vi "ROS_Master_getPublishedTopicsReply.vi"(2 "Subgraph":string, 3 "ROS_Master":T1) -> (0 "XML":string)   [LabVIEW 2014]
doc: "Returns the XML reply for a published topic"
uses:
  <userlib>/ROS for LabVIEW Software/ROS/Code/ROS_Master/ROS_Master.ctl
  <userlib>/ROS for LabVIEW Software/ROS/Code/ROS_Master/ROS_Topic.ctl
  <userlib>/ROS for LabVIEW Software/ROS/Code/ROS_Master/ROS_Node.ctl
  <userlib>/ROS for LabVIEW Software/ROS/Code/ROS_Master/ROS_Service.ctl
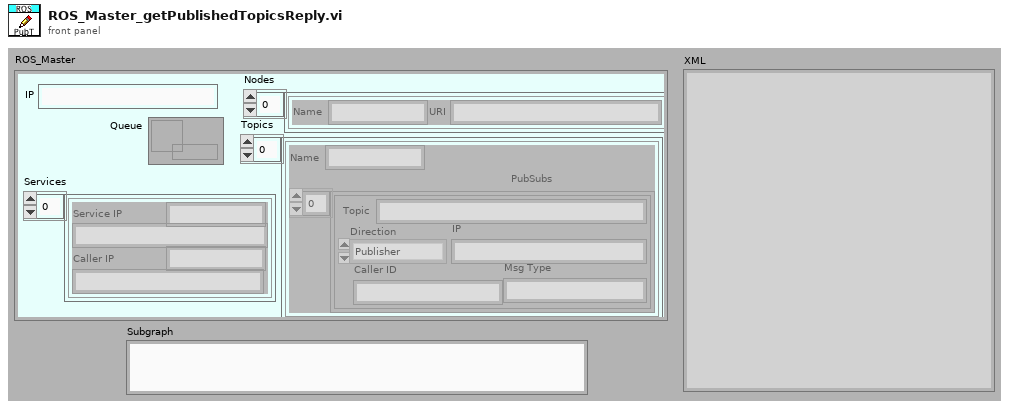
[diagram p1: front panel]
types:
  T1 = typedef "ROS_Master.ctl" = cluster{"IP":string, "Topics":cluster{"Name":string, "PubSubs":T2[]}[], "Nodes":T3[], "Services":T4[], "Queue":refnum<queue>}
  T2 = typedef "ROS_Topic.ctl" = cluster{"Caller ID":string, "IP":string, "Msg Type":string, "Direction":enum16{"Publisher", "Subscriber"}, "Topic":string}
  T3 = typedef "ROS_Node.ctl" = cluster{"Name":string, "URI":string}
  T4 = typedef "ROS_Service.ctl" = cluster{"Service":string, "Service IP":string, "Caller IP":string, "Caller ID":string}
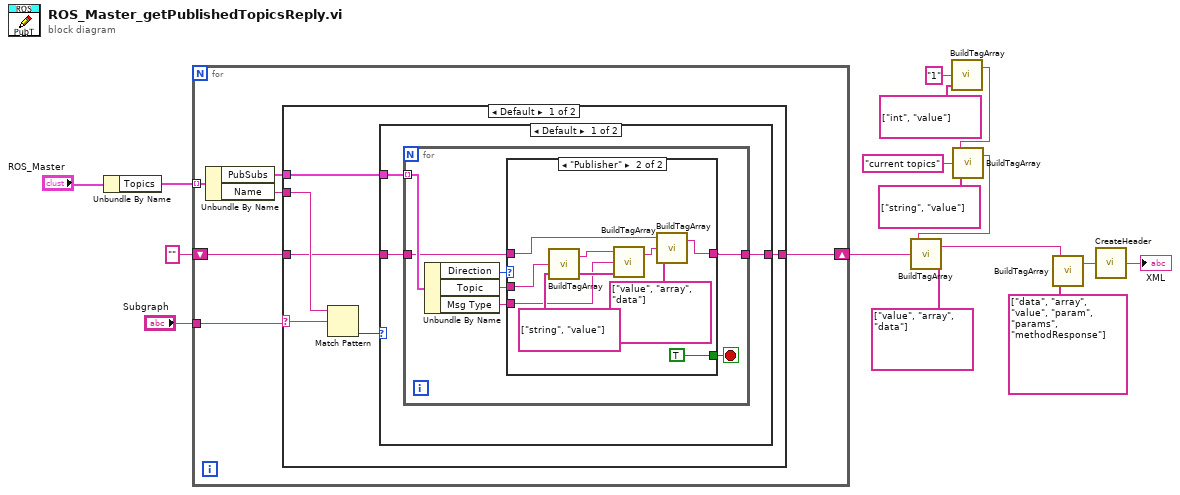
[diagram p0: block diagram]
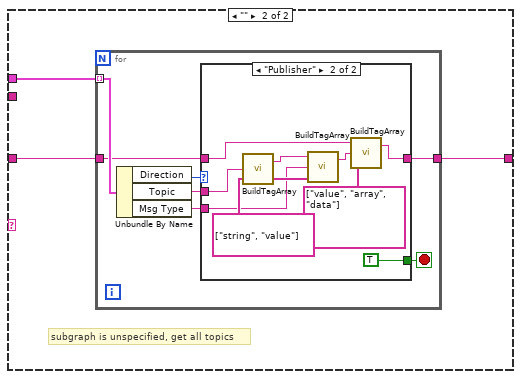
[diagram p4: hidden frame]
diagram:
  n1 = Unbundle By Name("ROS_Master") -> ("Topics"=w16:cluster{"Name":string, "PubSubs":T2[]}[])
  n2 = for {
    tunnel: w16 -> [w20] mode=indexing
    tunnel: "Subgraph" -> [w22]
    shift-right: [w17] -> w7
    shift-left: "" ("tag") -> [w18]
    n3 = Unbundle By Name(w20) -> ("PubSubs"=w19:T2[], "Name"=w21:string)
    n4 = case shown="Default" w22 {
      selector: w22 -> [w27 _]
      tunnel: w21 -> [w28 _]
      tunnel: w19 -> [w25 w52]
      tunnel: w18 -> [w24 w51]
      tunnel: [w23 w50] -> w17
      frame Default {
        n5 = Match Pattern(string=w28, regular expression=w27) -> (offset past match=w26:i32)  [unwired: 1 in, 3 out]
        n6 = case shown="Default" w26 {
          tunnel: w25 -> [w31 _]
          tunnel: w24 -> [w30 w49]
          tunnel: [w29 w49] -> w23
          frame Default {
            n7 = for {
              tunnel: w31 -> [w38] mode=indexing
              tunnel: w30 -> [w37]
              tunnel: [w36] -> w29
              stop <- w32 stop-if-true
              n8 = Unbundle By Name(w38) -> ("Direction"=w35:enum16{"Publisher", "Subscriber"}, "Topic"=w34:string, "Msg Type"=w33:string)
              n9 = case shown="\"Publisher\"" w35 {
                tunnel: [_ TRUE] -> w32
                tunnel: w34 -> [_ w46]
                tunnel: w33 -> [_ w44]
                tunnel: w37 -> [w39 w41]
                tunnel: [w39 w40] -> w36
                frame Default {
                }
                frame "Publisher" {
                  w47 = string[] ["string", "value"] ("tags")
                  n10 = call <userlib>:"BuildTagArray.vi"("tags"=w47, "value"=w46) -> ("string out"=w45:string)  [unwired: 2 in]
                  n11 = call <userlib>:"BuildTagArray.vi"("tags"=w47, "value"=w44, "string in"=w45) -> ("string out"=w43:string)  [unwired: 1 in]
                  n12 = call <userlib>:"BuildTagArray.vi"("tags"=string[] ["value", "array", "data"], "value"=w43, "string in"=w41) -> ("string out"=w40:string)  [unwired: 1 in]
                }
              }
            }
          }
          frame -1 {
            # "subgraph doesn't match topic"
          }
        }
      }
      frame "" {
        # "subgraph is unspecified, get all topics"
        n13 = for {
          tunnel: w52 -> [w59] mode=indexing
          tunnel: w51 -> [w54]
          tunnel: [w53] -> w50
          stop <- w57 stop-if-true
          n14 = Unbundle By Name(w59) -> ("Direction"=w58:enum16{"Publisher", "Subscriber"}, "Topic"=w56:string, "Msg Type"=w55:string)
          n15 = case shown="\"Publisher\"" w58 {
            tunnel: [_ TRUE] -> w57
            tunnel: w56 -> [_ w67]
            tunnel: w55 -> [_ w65]
            tunnel: w54 -> [w60 w62]
            tunnel: [w60 w61] -> w53
            frame Default {
            }
            frame "Publisher" {
              w68 = string[] ["string", "value"] ("tags")
              n16 = call <userlib>:"BuildTagArray.vi"("tags"=w68, "value"=w67) -> ("string out"=w66:string)  [unwired: 2 in]
              n17 = call <userlib>:"BuildTagArray.vi"("tags"=w68, "value"=w65, "string in"=w66) -> ("string out"=w64:string)  [unwired: 1 in]
              n18 = call <userlib>:"BuildTagArray.vi"("tags"=string[] ["value", "array", "data"], "value"=w64, "string in"=w62) -> ("string out"=w61:string)  [unwired: 1 in]
            }
          }
        }
      }
    }
  }
  n19 = call <userlib>:"BuildTagArray.vi"("tags"=string[] ["int", "value"], "value"="1") -> ("string out"=w9:string)  [unwired: 2 in]
  n20 = call <userlib>:"BuildTagArray.vi"("tags"=string[] ["string", "value"], "value"="current topics", "string in"=w9) -> ("string out"=w6:string)  [unwired: 1 in]
  n21 = call <userlib>:"BuildTagArray.vi"("tags"=string[] ["value", "array", "data"], "value"=w7, "string in"=w6) -> ("string out"=w5:string)  [unwired: 1 in]
  n22 = call <userlib>:"BuildTagArray.vi"("tags"=string[] ["data", "array", "value", "param", "params", "methodResponse"], "value"=w5) -> ("string out"=w3:string)  [unwired: 2 in]
  n23 = call <userlib>:"CreateHeader.vi"("Content"=w3) -> ("XML"=→"XML":string)
